vi "Data_Convert.vi"(0 "Data Type":u8, 1 "Array":u8[](array[numeric])) -> (2 "D Int out":i32, 3 "D Float out":sgl, 4 "Int_F":bool)   [LabVIEW 2017]
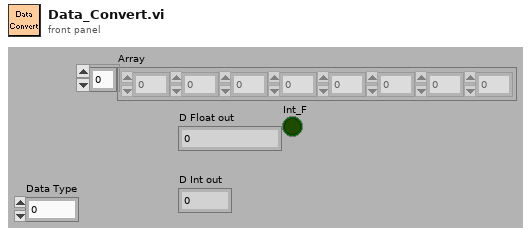
[diagram p1: front panel]
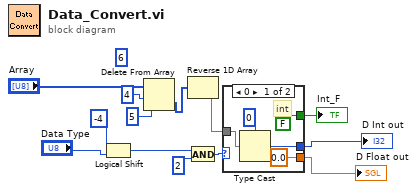
[diagram p0: block diagram]
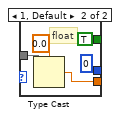
[diagram p2: hidden frame]
diagram:
  (unwired) 6 ("length")
  n1 = Logical Shift(y=i8 -4, x="Data Type") -> (x << y=w5:u8)
  n2 = Delete From Array(array="Array", length=4, index=5) -> (deleted portion=w3:u8[])  [unwired: 1 out]
  n3 = Reverse 1D Array(array=w3) -> (reversed array=w2:u8[])
  n4 = And(x=w5, y=u8 2) -> (x .and. y?=w8:u8)
  n5 = case shown="0" w8 {
    tunnel: w2 -> [w17 w22]
    tunnel: [w16 0 ("Numeric 2")] -> w12
    tunnel: [sgl 0.0 ("Numeric 2") w21] -> w13
    tunnel: [FALSE TRUE] -> w1
    frame 0 {
      # "int"
      n6 = Type Cast(type=0 ("Numeric 2"), x=w17) -> (*(type *) &x=w16:i32)
    }
    frame 1, Default {
      # "float"
      n7 = Type Cast(type=sgl 0.0 ("Numeric 2"), x=w22) -> (*(type *) &x=w21:sgl)
    }
  }
  "D Float out" <- w13
  "D Int out" <- w12
  "Int_F" <- w1
